vi "JSON_reader.vi"() -> ()   [LabVIEW 2016]
doc: "Grab the .project8_authentications.json file in the home and read the AMQP credentials."
uses:
  global/AMQP_credentials.vi
panel:
  out "Path":path
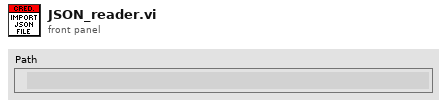
[diagram p1: front panel]
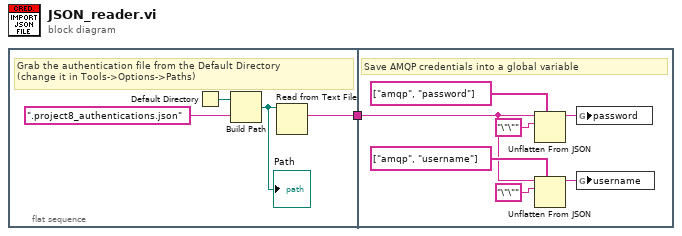
[diagram p0: block diagram]
diagram:
  n1 = flat-sequence {
    tunnel: [w2] -> w1
    tunnel: w1 -> [w6]
    frame #0 {
      # "Grab the authentication file from the Default Directory\n(change it in Tools->Options->Paths)"
      n2 = Default Directory() -> (w3:path)
      n3 = Build Path(base path=w3, name or relative path=".project8_authentications.json") -> (appended path=w5:path)
      "Path" <- w5
      n4 = Read from Text File(file (use dialog)=w5) -> (text=w2:string)  [unwired: 3 in, 3 out]
    }
    frame #1 {
      # "Save AMQP credentials into a global variable"
      n5 = Unflatten From JSON(path=string[] ["amqp", "password"], JSON string=w6, type and defaults="\"\"") -> (value=w7:string)  [unwired: 4 in, 1 out]
      n6 = Unflatten From JSON(path=string[] ["amqp", "username"], JSON string=w6, type and defaults="\"\"") -> (value=w10:string)  [unwired: 4 in, 1 out]
      n7 = global write "AMQP_credentials.vi" "password"(w7) -> ()
      n8 = global write "AMQP_credentials.vi" "username"(w10) -> ()
    }
  }
